vi "Fetch_original_waveform_timing.vi"(8 "error in (no error)":errorcluster, 9 "Maximum Time (10000ms)":u32=10000, 11 "VISA resource name":refnum<visa-resource-name>) -> (0 "error out":errorcluster, 1 "low level read time":u32, 2 "Waveform Data":waveform(dbl)(graph)={"t0"=timestamp(3.694502999999883e-07 s since 1904-01-01), "dt"=5e-07, "Y"=array[10000 elements]}, 3 "VISA resource name out":refnum<visa-resource-name>, 4 "curve and length command":u32)   [LabVIEW 2011]
doc: "Returns the waveform that an oscilloscope acquires for a channel you specify. An acquisition that you initiate before calling this VI generates the waveform.\n\nYou first enable channels with the Configure Channel VI. Then you use the Initiate VI to start an acquisition on the enabled channels. An oscilloscope concurrently acquires waveforms for these channels. You must call the Fetch Waveform VI separately to obtain waveforms for each enabled channel. However, you also can call the Read Waveform VI instead of using the above low-level VIs.\n\n<B>Note:</B> Use the Fetch Waveform VI only with other low-level VIs, such as the Initiate VI, the Abort VI, and the Fetch Waveform Measurement VI. High-level VIs such as the Read Waveform VI automatically incorporate the functions of the Initiate VI and the Fetch Waveform VI. The Fetch Waveform VI does not check the status of an instrument."
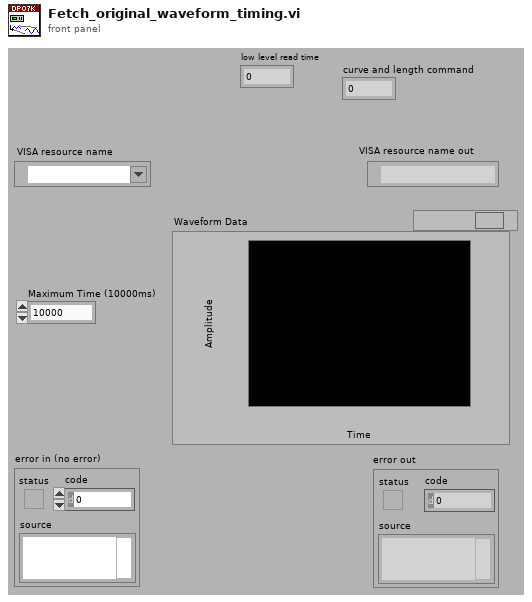
[diagram p1: front panel]
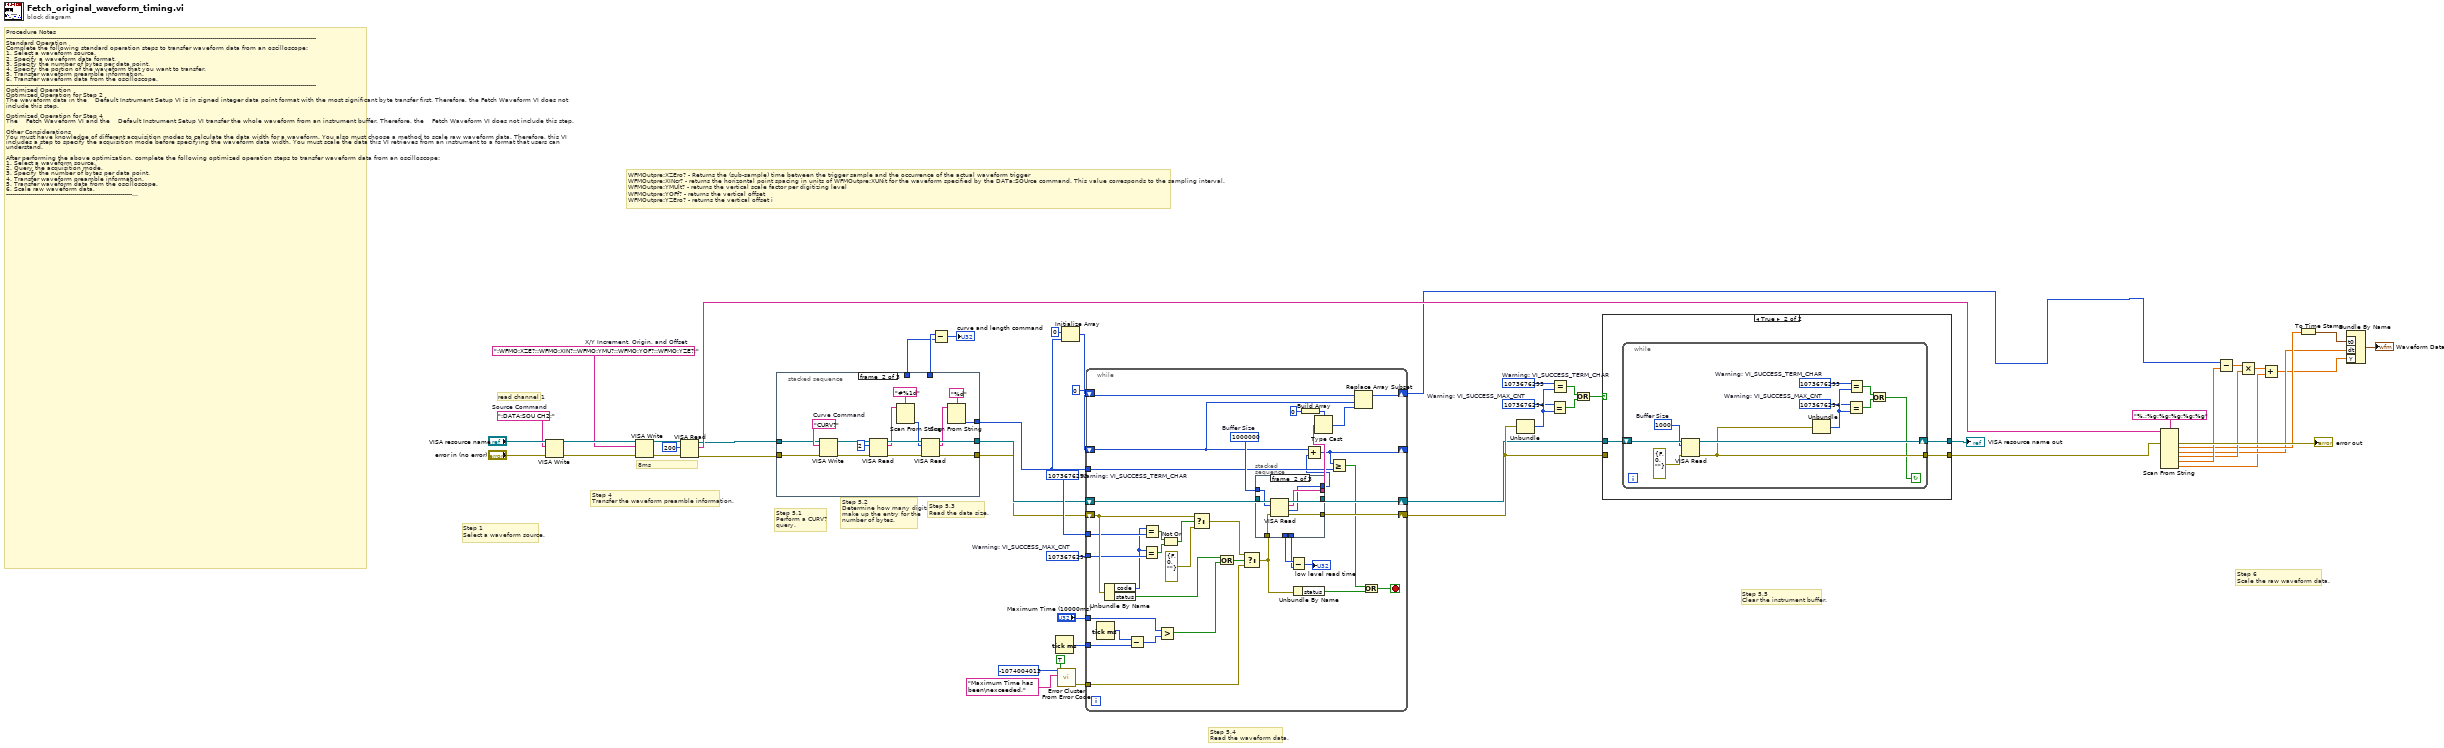
[diagram p0: block diagram]
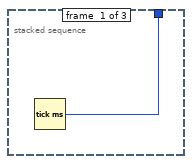
[diagram p2: hidden frame]
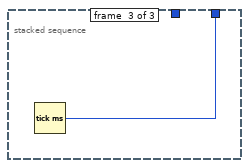
[diagram p3: hidden frame]
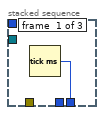
[diagram p5: hidden frame]
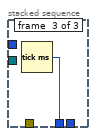
[diagram p6: hidden frame]
diagram:
  w7 = ":WFMO:XZE?;:WFMO:XIN?;:WFMO:YMU?;:WFMO:YOF?;:WFMO:YZE?;"  # X/Y Increment, Origin, and Offset
  w37 = 1073676294  # Warning: VI_SUCCESS_MAX_CNT
  w38 = 1073676293  # Warning: VI_SUCCESS_TERM_CHAR
  w41 = 1073676294  # Warning: VI_SUCCESS_MAX_CNT
  w40 = 1073676293  # Warning: VI_SUCCESS_TERM_CHAR
  w11 = ":DATA:SOU CH2;"  # Source Command
  # "Step 5.1      \nPerform a CURV?\nquery."
  # "8ms"
  # "read channel 1"
  # "WFMOutpre:XZEro? - Returns the (sub-sample) time between the trigger sample and the occurrence of the actual waveform trigger\nWFMOutpre:XINcr? - returns the horizontal point spacing in units of WFMOutpre:XUNit for the waveform specified by the DATa:SOUrce command. This value corresponds to the sampling interval.\nWFMOutpre:YMUlt? - returns the vertical scale factor per digitizing level \nWFMOutpre:YOFf? - returns the vertical offset \nWFMOutpre:YZEro? - returns the vertical offset i"
  # "Step 1       \nSelect a waveform source."
  # "Step 6    \nScale the raw waveform data."
  # "Step 5.5    \nClear the instrument buffer."
  # "Step 5.4   \nRead the waveform data."
  # "Step 5.3      \nRead the data size."
  # "Step 5.2      \nDetermine how many digits\nmake up the entry for the \nnumber of bytes."
  # "Step 4\nTransfer the waveform preamble information."
  # "Procedure Notes\n-----------------------------------------------------------------------------------------------------------------------------------------------------------\nStandard Operation\nComplete the following standard operation steps to transfer waveform data from an oscilloscope:\n1. Select a waveform source.\n2. Specify a waveform data format.\n3. Specify the number of bytes per data point.\n4. Specify the portion of the waveform that you want to transfer.\n5. Transfer waveform preamble information.\n6. Transfer waveform data from the oscilloscope.\n-----------------------------------------------------------------------------------------------------------------------------------------------------------\nOptimized Operation\nOptimized Operation for Step 2\nThe waveform data in the    Default Instrument Setup VI is in signed integer data point format with the most significant byte transfer first. Therefore, the Fetch Waveform VI does not include this step.\n\nOptimized Operation for Step 4 \nThe    Fetch Waveform VI and the    Default Instrument Setup VI transfer the whole waveform from an instrument buffer. Therefore, the    Fetch Waveform VI does not include this step.\n\nOther Considerations\nYou must have knowledge of different acquisition modes to calculate the data width for a waveform. You also must choose a method to scale raw waveform data. Therefore, this VI includes a step to specify the acquisition mode before specifying the waveform data width. You must scale the data this VI retrieves from an instrument to a format that users can understand.\n\nAfter performing the above optimization, complete the following optimized operation steps to transfer waveform data from an oscilloscope:\n1. Select a waveform source.\n2. Query the acquisition mode.\n3. Specify the number of bytes per data point.\n4. Transfer waveform preamble information.\n5. Transfer waveform data from the oscilloscope.\n6. Scale raw waveform data.\n-----------------------------------------------------------------------------------------------------------------------------------------------------------\nDetailed Steps\nThe following steps detail the behavior of this VI:\n1. Select a waveform source. \n2. Query and determine the acquisition mode. A correct determination is critical to steps 3 and 6.\n    -----------------------------------------------\n    Acquisition Mode |  Data Width   \n    -----------------------------------------------\n    Normal                       |   1                      \n    -----------------------------------------------\n    Peak Detect               |   1                      \n    -----------------------------------------------\n    Hi Res                        |   2                      \n    -----------------------------------------------\n    Envelope                   |   1                      \n    ----------------------------------------------- \n    Average                    |   2                      \n    -----------------------------------------------\n3. Specify the number of bytes per data point. For the Hi Res or Average acquisition modes, set the data width to 2. For all other acquisition modes, set the data width to 1.\n4. Transfer the waveform preamble information. Necessary preamble information includes XZero, XIncrement, YMultiplier, YOffset, and YZero. This VI uses XZero and XIncrement to configure the x-axis of output waveforms and uses YMultiplier, YOffset, and YZero to scale data values. This VI then parses the return string of the preamble query in step 6.\n5. Transfer waveform data from the oscilloscope.\n    5.1 Perform a CURV? query.\n    5.2 Determine how many digits make up the entry for the number of bytes.\n    5.3 Read the data size.\n    5.4 Call the VISA Read VI repeatedly with a buffer size of 10000 until you obtain as much data as the data size specifies. Use      an 8-bit array to store the raw waveform data you obtain. \n    5.5 Continue reading the data remaining in the instrument buffer until the buffer is empty.\n6. Scale the raw waveform data.\n    6.1 Cast the waveform data to a 16-bit array if the data width is 2. Split the waveform data into a minimum and a maximum data array if the acquisition mode is Peak Detect or Envelope. This VI skips this step if the data width is 1.\n    6.2 Parse the preamble information.\n    6.3 Scale the waveform data according to the following formula:\n          Data_Value_in_units = (Raw_Data_Value - YOffset) * YMultiplier + YZero\n          The resulting waveform data has a unit of volts.\n    6.4 Build a waveform graph."
  n1 = VISA Write(VISA resource name="VISA resource name", write buffer=w11, error in (no error)="error in (no error)") -> (VISA resource name out=w13:refnum<visa-resource-name>, error out=w12:errorcluster)  [unwired: 1 out]
  n2 = VISA Write(VISA resource name=w13, write buffer=w7, error in (no error)=w12) -> (VISA resource name out=w9:refnum<visa-resource-name>, error out=w8:errorcluster)  [unwired: 1 out]
  n3 = VISA Read(VISA resource name=w9, byte count=u32 200, error in (no error)=w8) -> (VISA resource name out=w6:refnum<visa-resource-name>, read buffer=w52:string, error out=w5:errorcluster)  [unwired: 1 out]
  n4 = stacked-sequence {
    tunnel: [_ w69 _] -> w48
    tunnel: [_ w68 _] -> w26
    tunnel: [_ w67 _] -> w25
    tunnel: w6 -> [_ w55 _]
    tunnel: w5 -> [_ w54 _]
    tunnel: [_ _ w70] -> w4
    tunnel: [w53 _ _] -> w3
    frame #0 {
      n5 = Tick Count (ms)() -> (millisecond timer value=w53:u32)
    }
    frame #1 {
      w66 = "CURV?"  # Curve Command
      n6 = VISA Write(VISA resource name=w55, write buffer=w66, error in (no error)=w54) -> (VISA resource name out=w56:refnum<visa-resource-name>, error out=w65:errorcluster)  [unwired: 1 out]
      n7 = VISA Read(VISA resource name=w56, byte count=u32 2, error in (no error)=w65) -> (VISA resource name out=w62:refnum<visa-resource-name>, read buffer=w60:string, error out=w61:errorcluster)  [unwired: 1 out]
      n8 = Scan From String(format string="#%1d", input string=w60) -> (output 1=w59:i32)  [unwired: 3 in, 3 out]
      n9 = VISA Read(VISA resource name=w62, byte count=w59, error in (no error)=w61) -> (VISA resource name out=w68:refnum<visa-resource-name>, read buffer=w57:string, error out=w67:errorcluster)  [unwired: 1 out]
      n10 = Scan From String(format string="%d", input string=w57) -> (output 1=w69:i32)  [unwired: 3 in, 3 out]
    }
    frame #2 {
      n11 = Tick Count (ms)() -> (millisecond timer value=w70:u32)
    }
  }
  n12 = Subtract(x=w4, y=w3) -> (x-y=→"curve and length command":u32)
  n13 = Tick Count (ms)() -> (millisecond timer value=w18:u32)
  n14 = call <vilib>:"Error Cluster From Error Code.vi"("show call chain? (False)"=TRUE, "error message (\"\")"="Maximum Time has been\nexceeded." ("error message (\"\")"), "error code (0)"=-1074004013) -> ("error out"=w16:errorcluster)  [unwired: 6 in]
  n15 = Initialize Array(i8 0 ("element"), w48) -> (w46:i8[])
  n16 = while {
    shift-right: [w106] -> w14
    shift-left: w26 -> [w108]
    shift-right: [w105] -> w15
    shift-left: w25 -> [w95]
    shift-right: [w101] -> w1
    shift-left: w46 -> [w102]
    tunnel: w48 -> [w99]
    shift-right: [w96] -> _
    shift-left: 0 -> [w97]
    tunnel: w38 -> [w94]
    tunnel: w37 -> [w93]
    tunnel: w18 -> [w87]
    tunnel: "Maximum Time (10000ms)" -> [w86]
    tunnel: w16 -> [w81]
    stop <- w77 stop-if-true
    w107 = 1000000  # Buffer Size
    n17 = Tick Count (ms)() -> (millisecond timer value=w88:u32)
    n18 = Unbundle By Name(w95) -> ("code"=w92:i32, "status"=w80:bool)
    n19 = Subtract(x=w88, y=w87) -> (x-y=w85:u32)
    n20 = Equal?(x=w92, y=w93) -> (x = y?=w90:bool)
    n21 = Equal?(x=w92, y=w94) -> (x = y?=w91:bool)
    n22 = Greater?(x=w86, y=w85) -> (0:w79:bool)
    n23 = Not Or(1:w90, 2:w91) -> (0:w89:bool)
    n24 = Select(t=w95, s=w89, f=errorcluster {"status"=FALSE, "code"=0, "source"=""} ("error in (no error)")) -> (s? t:f=w82:errorcluster)
    n25 = Or(x=w80, y=w79) -> (x .or. y?=w83:bool)
    n26 = Select(t=w82, s=w83, f=w81) -> (s? t:f=w76:errorcluster)
    n27 = stacked-sequence {
      tunnel: w108 -> [_ w116 _]
      tunnel: w107 -> [_ w115 _]
      tunnel: [_ w114 _] -> w106
      tunnel: [_ w113 _] -> w105
      tunnel: [_ w112 _] -> w100
      tunnel: [_ w111 _] -> w74
      tunnel: w76 -> [_ w110 _]
      tunnel: [_ _ w117] -> w73
      tunnel: [w109 _ _] -> w72
      frame #0 {
        n28 = Tick Count (ms)() -> (millisecond timer value=w109:u32)
      }
      frame #1 {
        n29 = VISA Read(VISA resource name=w116, byte count=w115, error in (no error)=w110) -> (VISA resource name out=w114:refnum<visa-resource-name>, read buffer=w112:string, return count=w111:u32, error out=w113:errorcluster)
      }
      frame #2 {
        n30 = Tick Count (ms)() -> (millisecond timer value=w117:u32)
      }
    }
    n31 = Subtract(x=w73, y=w72) -> (x-y=→"low level read time":u32)
    n32 = Unbundle By Name(w76) -> ("status"=w75:bool)
    n33 = Build Array(i8 0) -> (w104:i8[])
    n34 = Add(x=w97, y=w74) -> (x+y=w96:u32)
    n35 = Type Cast(type=w104, x=w100) -> (*(type *) &x=w98:i8[])
    n36 = Greater Or Equal?(x=w96, y=w99) -> (x >= y?=w78:bool)
    n37 = Replace Array Subset(array=w102, new element=w98, index=w97) -> (w101:i8[])
    n38 = Or(x=w78, y=w75) -> (x .or. y?=w77:bool)
  }
  n39 = Unbundle(w15) -> ("code"=w42:i32)  [unwired: 2 out]
  n40 = Equal?(x=w41, y=w42) -> (x = y?=w44:bool)
  n41 = Equal?(x=w40, y=w42) -> (x = y?=w45:bool)
  n42 = Or(x=w45, y=w44) -> (x .or. y?=w43:bool)
  n43 = case shown="True" w43 {
    tunnel: w14 -> [w119 w122]
    tunnel: w15 -> [w118 _]
    tunnel: [w119 w121] -> w49
    tunnel: [w118 w120] -> w51
    frame False {
    }
    frame True {
      n44 = while {
        shift-right: [w132] -> w121
        shift-left: w122 -> [w133]
        tunnel: [w125] -> w120
        stop <- w124 continue-if-true
        w127 = 1073676294  # Warning: VI_SUCCESS_MAX_CNT
        w126 = 1073676293  # Warning: VI_SUCCESS_TERM_CHAR
        w131 = u32 1000  # Buffer Size
        n45 = VISA Read(VISA resource name=w133, byte count=w131, error in (no error)=errorcluster {"status"=FALSE, "code"=0, "source"=""}) -> (VISA resource name out=w132:refnum<visa-resource-name>, error out=w125:errorcluster)  [unwired: 2 out]
        n46 = Unbundle(w125) -> ("code"=w128:i32)  [unwired: 2 out]
        n47 = Equal?(x=w127, y=w128) -> (x = y?=w129:bool)
        n48 = Equal?(x=w126, y=w128) -> (x = y?=w130:bool)
        n49 = Or(x=w130, y=w129) -> (x .or. y?=w124:bool)
      }
    }
  }
  "VISA resource name out" <- w49
  n50 = Scan From String(format string="%.;%g;%g;%g;%g;%g", input string=w52, error in=w51) -> (error out=→"error out":errorcluster, output 1=w29:dbl, output 2=w27:dbl, output 3=w33:dbl, output 4=w34:dbl, output 5=w23:dbl)  [unwired: 6 in, 2 out]
  n51 = Subtract(x=w1, y=w34) -> (x-y=w35:dbl[])
  n52 = Multiply(x=w35, y=w33) -> (x*y=w24:dbl[])
  n53 = Add(x=w24, y=w23) -> (x+y=w22:dbl[])
  n54 = To Time Stamp(1:w29) -> (0:w28:timestamp)
  n55 = Bundle By Name ("Build Waveform")("t0"=w28, "dt"=w27, "Y"=w22) -> (→"Waveform Data":waveform(dbl))  [unwired: 1 in]
